vi "sql testing.vi"() -> (3 "MAX Rejection ID":i32)   [LabVIEW 2017]
uses:
  <vilib>/addons/database/Connection.llb/Conn ObjectReference.ctl
  <vilib>/addons/database/Connection.llb/DB Tools Open Connec (Path).vi
  <vilib>/addons/database/Connection.llb/Conn Execute.vi
  <vilib>/addons/database/Recordset.llb/Rec Fetch Recordset Data (R).vi
  <vilib>/addons/database/Recordset.llb/Rec Destroy - Connection.vi
  <vilib>/addons/database/NI_Database_API.lvlib
panel:
  out "SHIFT":i32
  out "data":string
  out "recordset data":variant[][](array[variant])
  out "resulting string":string
  in  "Product code":string
  in  "REJECTION COUNT 2":i32
  out "REJ COUNT":i32
  out "error out 3":errorcluster
  out "Refnum out 2":T1
  in  "MAX BREAKDOWN ID 2":i32
  in  "Station":string
  in  "Current Shift":i32
  out "error out 2":errorcluster
  out "REJECTION COUNT":i32
  out "TABLE NAME":string
  out "error out":errorcluster
  # "Rejection check and add to DataBase"
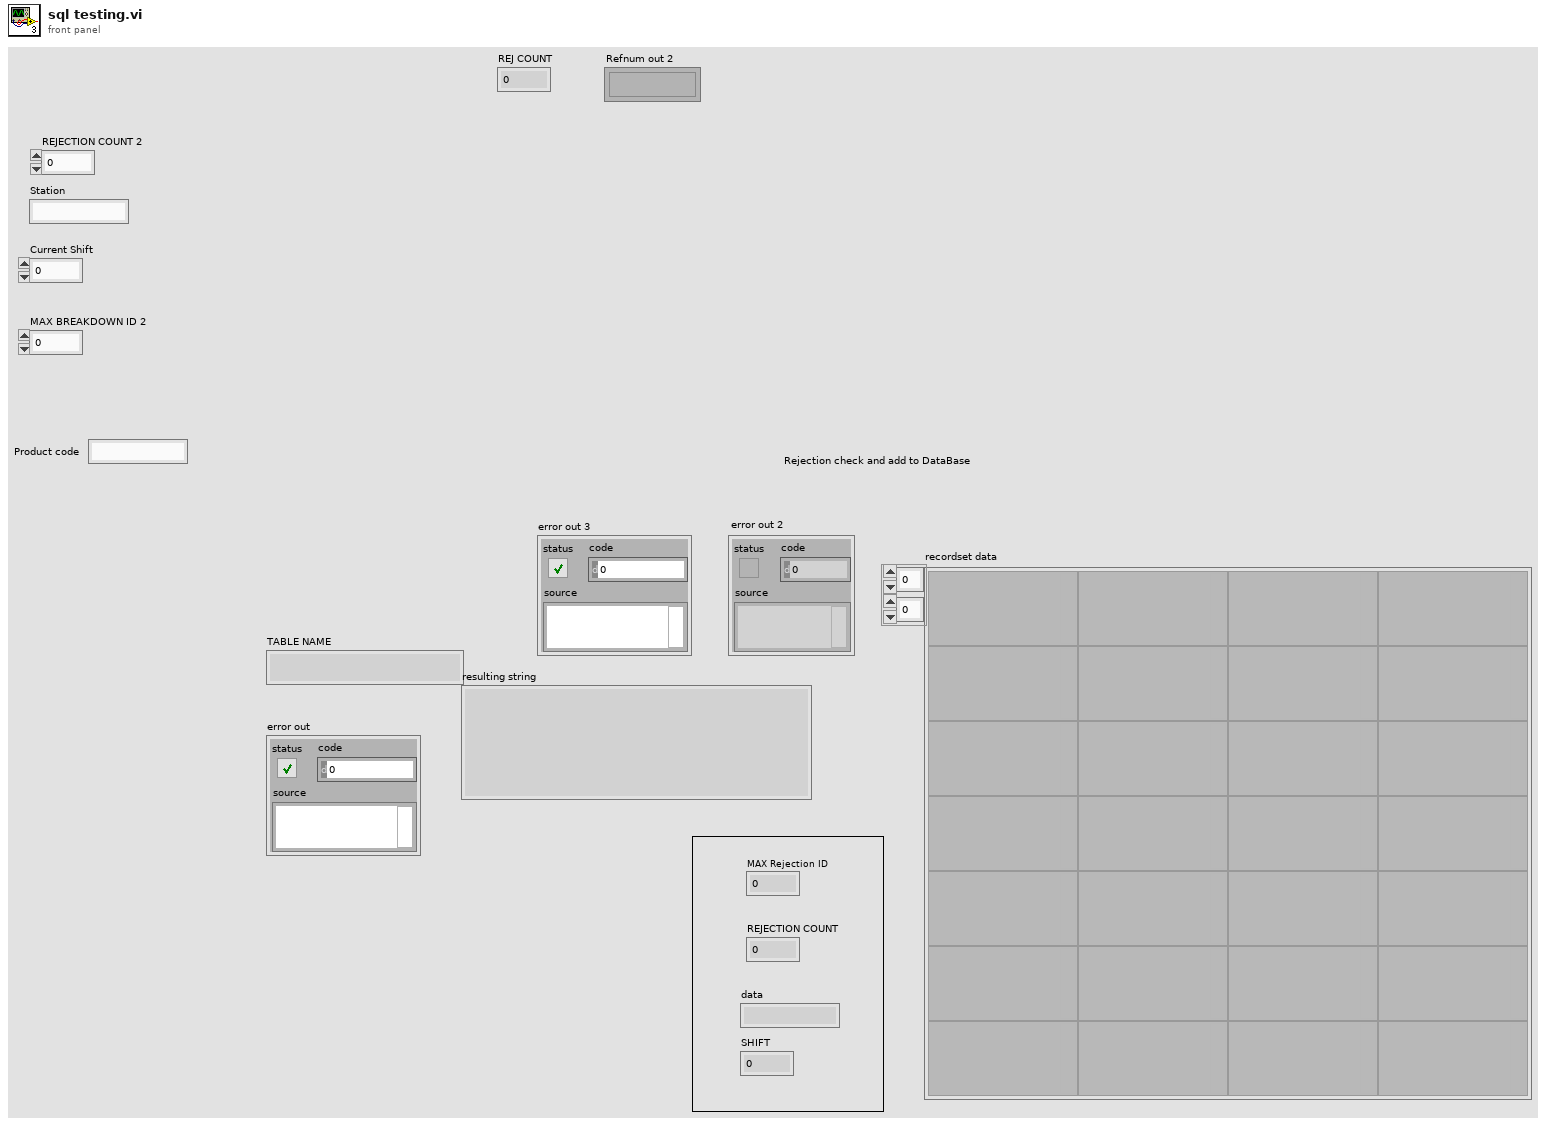
[diagram p1: front panel]
types:
  T1 = typedef "NI_Database_API.lvlib/Conn ObjectReference.ctl" = refnum<k1>
  T2 = typedef "NI_Database_API.lvlib/Rec ObjectReference.ctl" = refnum<k1>
  T3 = typedef "LVDateTimeRec.ctl" = cluster{"fractional second":dbl, "second":i32, "minute":i32, "hour":i32, "day of month":i32, "month":i32, "year":i32, "day of week":i32, "day of year":i32, "DST":i32}
  T4 = cluster{i32, "Station":string, i32, "Current Shift":i32, "date/time string":string, "Date String":string, "Product code":string}
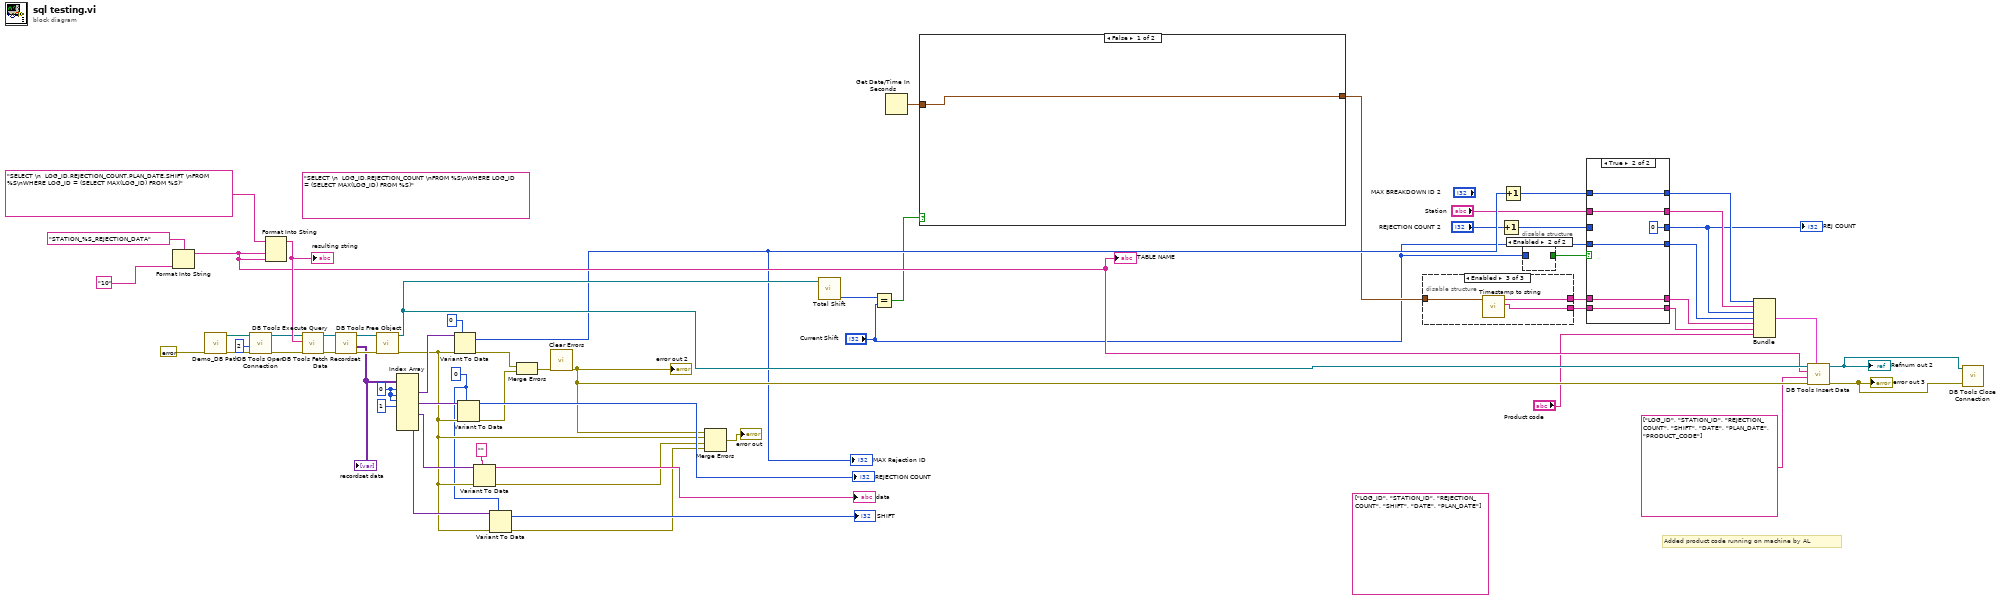
[diagram p0: block diagram]
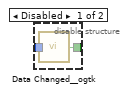
[diagram p2: hidden frame]
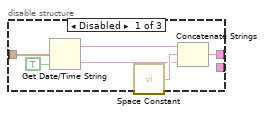
[diagram p3: hidden frame]
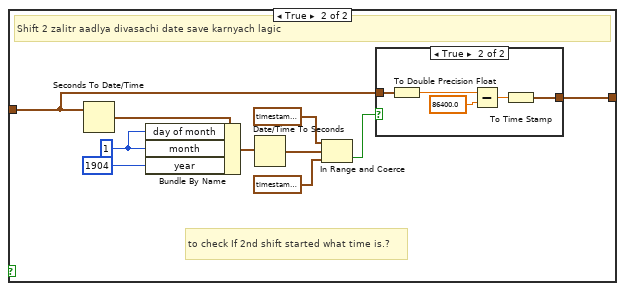
[diagram p5: hidden frame]
diagram:
  (unwired) string[] ["LOG_ID", "STATION_ID", "REJECTION_COUNT", "SHIFT", "DATE", "PLAN_DATE"] ("columns")
  (unwired) "SELECT \n  LOG_ID,REJECTION_COUNT \nFROM %S\nWHERE LOG_ID = (SELECT MAX(LOG_ID) FROM %S)" ("SQL query")
  w27 = 0
  w49 = 0 ("index (row)")
  # "Added product code running on machine by AL"
  n1 = Format Into String(format string="STATION_%S_REJECTION_DATA" ("SQL query"), "10" ("Station No.")) -> (resulting string=w35:string)  [unwired: 2 in, 1 out]
  "TABLE NAME" <- w35
  n2 = call "Demo_DB Path.vi"("error in"=errorcluster {"status"=FALSE, "code"=0, "source"=""} ("error constant")) -> ("error out"=w43:errorcluster, "DB Path"=w42:path)  [unwired: 9 in]
  n3 = call-poly <vilib>:"DB Tools Open Connection.vi"("error in (no error)"=w43, "connection timeout (15)"=2, "connection information"=w42) -> ("error out"=w39:errorcluster, "connection reference"=w38:T1)  [unwired: 5 in]
  n4 = Format Into String(format string="SELECT \n  LOG_ID,REJECTION_COUNT,PLAN_DATE,SHIFT \nFROM %S\nWHERE LOG_ID = (SELECT MAX(LOG_ID) FROM %S)" ("SQL query"), w35, w35) -> (resulting string=w54:string)  [unwired: 2 in, 1 out]
  "resulting string" <- w54
  n5 = call-poly <vilib>:"DB Tools Execute Query.vi"("error in (no error)"=w39, "SQL query"=w54, "connection reference"=w38) -> ("error out"=w58:errorcluster, "recordset reference"=w59:T2)  [unwired: 5 in]
  n6 = call-poly <vilib>:"DB Tools Fetch Recordset Data.vi"("error in (no error)"=w58, "recordset reference"=w59) -> ("error out"=w57:errorcluster, "recordset data"=w33:variant[][], "recordset reference out"=w60:T2)  [unwired: 3 in]
  "recordset data" <- w33
  n7 = call-poly <vilib>:"DB Tools Free Object.vi"("error in (no error)"=w57, "recordset reference"=w60) -> ("error out"=w28:errorcluster, "connection reference"=w36:T1)  [unwired: 8 in]
  n8 = Index Array(array=w33, index (row) #1=w49, index (col) #1=w49, index (row) #2=w49, index (col) #2=1 ("index (row)")) -> (element #1=w55:variant, element #2=w48:variant, element #3=w32:variant, element #4=w29:variant)  [unwired: 4 in]
  n9 = Variant To Data(error in=w28, type=0, Variant=w55) -> (data=w34:i32, error out=w61:errorcluster)
  "MAX Rejection ID" <- w34
  n10 = Variant To Data(error in=w28, type=w27, Variant=w48) -> (data=→"REJECTION COUNT":i32, error out=w45:errorcluster)
  n11 = Variant To Data(error in=w28, type="", Variant=w32) -> (data=→"data":string, error out=w25:errorcluster)
  n12 = Variant To Data(error in=w28, type=w27, Variant=w29) -> (data=→"SHIFT":i32, error out=w24:errorcluster)
  n13 = Merge Errors(w61, w45) -> (w46:errorcluster)
  n14 = call <vilib>:"Clear Errors.vi"("error in (no error)"=w46) -> ("error out"=w37:errorcluster)  [unwired: 5 in, 1 out]
  "error out 2" <- w37
  n15 = Merge Errors(w37, w28, w25, w24) -> (→"error out":errorcluster)
  n16 = call "Total Shift.vi"("connection reference"=w36) -> ("Total Shifts"=w11:i32)  [unwired: 9 in, 1 out]
  n17 = Equal?(x=w11, y="Current Shift") -> (x = y?=w12:bool)
  n18 = Get Date/Time In Seconds() -> (seconds since 1Jan1904=w10:timestamp)
  n19 = case shown="False" w12 {
    tunnel: w10 -> [w62 w63]
    tunnel: [w62 w64] -> w9
    frame False {
    }
    frame True {
      w69 = 1 ("day of month")
      # "to check If 2nd shift started what time is.?"
      # "Shift 2 zalitr aadlya divasachi date save karnyach lagic"
      n20 = Seconds To Date/Time(time stamp (now)=w63) -> (date time rec=w70:T3)  [unwired: 1 in]
      n21 = Bundle By Name(cluster=w70, "day of month"=w69, "month"=w69, "year"=1904) -> (w72:T3)
      n22 = Date/Time To Seconds(2:w72) -> (0:w68:timestamp)  [unwired: 1 in]
      n23 = In Range and Coerce(upper limit=timestamp(5399 s since 1904-01-01), x=w68, lower limit=timestamp(-19800 s since 1904-01-01)) -> (In Range?=w65:bool)  [unwired: 1 out]
      n24 = case shown="True" w65 {
        tunnel: [w73 w75] -> w64
        tunnel: w63 -> [w73 w74]
        frame False {
        }
        frame True {
          n25 = To Double Precision Float(number=w74) -> (double precision float=w78:dbl)
          n26 = Subtract(x=w78, y=86400.0) -> (x-y=w76:dbl)
          n27 = To Time Stamp(1:w76) -> (0:w75:timestamp)
        }
      }
    }
  }
  n28 = disable-structure shown="Enabled" {
    disable-tunnel: w9 -> [w84 w85 w88]
    disable-tunnel: [w80 w85 w87] -> w7
    disable-tunnel: [_ _ w86] -> w6
    frame Disabled {
      n29 = Get Date/Time String(seconds (now)=w84, want seconds? (F)=TRUE) -> (date string=w81:string, time string=w82:string)  [unwired: 1 in]
      n30 = call <vilib>:"Space Constant.vi"() -> ("String"=w83:string)
      n31 = Concatenate Strings(w81, w83, w82) -> (w80:string)
    }
    frame Disabled {
    }
    frame Enabled {
      n32 = call "Timestamp to string.vi"("time stamp"=w88) -> ("Date String"=w86:string, "date/time string"=w87:string)  [unwired: 8 in, 1 out]
    }
  }
  n33 = Increment(x="REJECTION COUNT 2") -> (x+1=w16:i32)
  n34 = Increment(x=w34) -> (x+1=w19:i32)
  n35 = disable-structure shown="Enabled" {
    disable-tunnel: [w90 _] -> w21
    disable-tunnel: "Current Shift" -> [w89 _]
    frame Disabled {
      n36 = call-poly <userlib>:"Data Changed__ogtk.vi"("I32"=w89) -> ("Changed"=w90:bool)
    }
    frame Enabled {
    }
  }
  n37 = case shown="True" w21 {
    tunnel: [w96 w102] -> w20
    tunnel: w19 -> [w96 w102]
    tunnel: [w95 w101] -> w18
    tunnel: "Station" -> [w95 w101]
    tunnel: [w94 0] -> w13
    tunnel: w16 -> [w94 _]
    tunnel: [w93 w100] -> w15
    tunnel: "Current Shift" -> [w93 w100]
    tunnel: [w92 w99] -> w14
    tunnel: w7 -> [w92 w99]
    tunnel: [w91 w97] -> w5
    tunnel: w6 -> [w91 w97]
    frame False {
    }
    frame True {
    }
  }
  "REJ COUNT" <- w13
  n38 = Bundle(w20, "Station"=w18, w13, "Current Shift"=w15, "date/time string"=w14, "Date String"=w5, "Product code"="Product code") -> (w23:T4)  [unwired: 1 in]
  n39 = call <vilib>:"DB Tools Insert Data.vi"("data"=w23, "error in (no error)"=w37, "columns"=string[] ["LOG_ID", "STATION_ID", "REJECTION_COUNT", "SHIFT", "DATE", "PLAN_DATE", "PRODUCT_CODE"], "table"=w35, "connection reference"=w36) -> ("error out"=w1:errorcluster, "connection reference out"=w2:T1)  [unwired: 5 in]
  "Refnum out 2" <- w2
  "error out 3" <- w1
  n40 = call <vilib>:"DB Tools Close Connection.vi"("error in (no error)"=w1, "connection reference"=w2) -> ()  [unwired: 5 in, 1 out]
